vi "WriteI64.vi"(10 "Data":i64, 11 "Address":u32) -> ()   [LabVIEW 2016]
uses:
  <vilib>/rvi/Memory/Memory_Emulation/nirvimemoryFastEmulation.vi
  <vilib>/rvi/Memory/Memory_Emulation/nirvimemoryEmulation.vi
  <vilib>/rvi/Emulation/niFpgaEmulationIsFPGAContextNoSignature.vi
  <vilib>/rvi/DataTransferAndStorage/Container/Common/niFpgaContainerGetUniqueNameForEmu.vi
  <vilib>/rvi/Emulation/niFpgaProcessEmulError.vi
  <vilib>/rvi/Emulation/niFpgaSctlEmulationGetInTimedLoop.vi
  <vilib>/rvi/errors/nirviReportUnexpectedCaseInternalError (U32).vi
  <vilib>/rvi/DataTransferAndStorage/Container/Common/niFpgaContainerExecOnDevCompGetState.vi
  <vilib>/rvi/Memory/Memory_Emulation/niFpgaMemoryEmulationCacheClearOnFirstRun.vi
  <vilib>/rvi/Memory/Memory_Emulation/nirvimemoryEmulationManagerCache_MakeExclusive.vi
  <vilib>/rvi/Memory/Memory_Emulation/niFpgaMemoryEmulationValidateCache.vi
  <vilib>/rvi/Memory/Memory_Emulation/nirvimemoryEmulationManagerCache_InsertValue.vi
  <vilib>/Utility/error.llb/Clear Errors.vi
  <vilib>/rvi/Memory/Memory_Emulation/nirvimemoryEmulationManagerCache_ReleaseExclusive.vi
  <vilib>/rvi/Memory/Memory_Emulation/nirvimemoryEmulationManagerCache_GetValue.vi
  <vilib>/rvi/Memory/Memory_Emulation/nirvimemoryEmulationManagerCache_SetValue.vi
  <vilib>/rvi/Emulation/niFpgaSctlEmulationResourceMgr.vi
  <vilib>/rvi/DataTransferAndStorage/Container/XNode/niFpgaContainer.xnode
  <vilib>/rvi/Memory/Memory_Emulation/niFpgaMemoryEmulationRefIn.vi
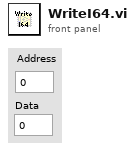
[diagram p1: front panel]
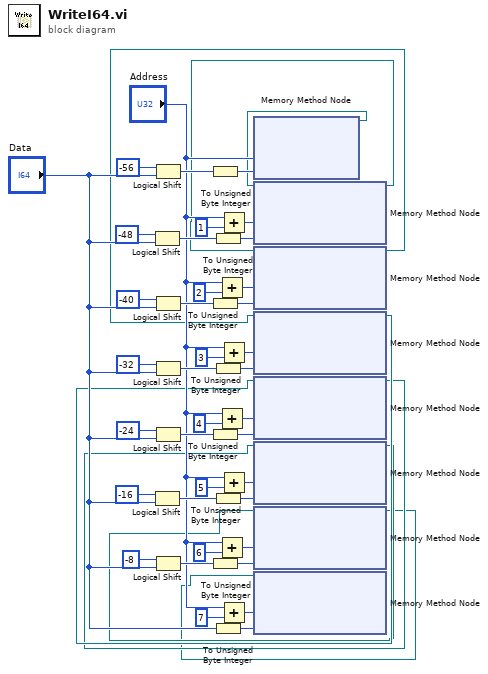
[diagram p0: block diagram]
diagram:
  n1 = Logical Shift(y=i16 -48, x="Data") -> (x << y=w30:i64)
  n2 = Logical Shift(y=i16 -16, x="Data") -> (x << y=w29:i64)
  n3 = Logical Shift(y=i16 -56, x="Data") -> (x << y=w41:i64)
  n4 = Logical Shift(y=i16 -40, x="Data") -> (x << y=w38:i64)
  n5 = Logical Shift(y=i16 -32, x="Data") -> (x << y=w12:i64)
  n6 = Logical Shift(y=i16 -24, x="Data") -> (x << y=w18:i64)
  n7 = Logical Shift(y=i16 -8, x="Data") -> (x << y=w21:i64)
  n8 = To Unsigned Byte Integer(number=w41) -> (unsigned 8bit integer=w42:u8)
  n9 = To Unsigned Byte Integer(number=w38) -> (unsigned 8bit integer=w37:u8)
  n10 = To Unsigned Byte Integer(number=w18) -> (unsigned 8bit integer=w17:u8)
  n11 = To Unsigned Byte Integer(number=w21) -> (unsigned 8bit integer=w22:u8)
  n12 = To Unsigned Byte Integer(number=w30) -> (unsigned 8bit integer=w40:u8)
  n13 = To Unsigned Byte Integer(number=w12) -> (unsigned 8bit integer=w39:u8)
  n14 = To Unsigned Byte Integer(number=w29) -> (unsigned 8bit integer=w19:u8)
  n15 = To Unsigned Byte Integer(number="Data") -> (unsigned 8bit integer=w20:u8)
  n16 = Add(x="Address", y=u32 2) -> (x+y=w32:u32)
  n17 = Add(x="Address", y=u32 4) -> (x+y=w10:u32)
  n18 = Add(x="Address", y=u32 6) -> (x+y=w27:u32)
  n19 = Add(x="Address", y=u32 1) -> (x+y=w45:u32)
  n20 = Add(x="Address", y=u32 3) -> (x+y=w34:u32)
  n21 = Add(x="Address", y=u32 5) -> (x+y=w14:u32)
  n22 = Add(x="Address", y=u32 7) -> (x+y=w25:u32)
  n23 = xnode ("Memory Method Node")("Address"="Address", "Data"=w42) -> ("Memory Out"=w7:refnum<k21>)  [unwired: 1 in]
  n24 = xnode ("Memory Method Node")("Address"=w45, "Data"=w40, "Memory In"=w7) -> ("Memory Out"=w6:refnum<k21>)
  n25 = xnode ("Memory Method Node")("Address"=w32, "Data"=w37, "Memory In"=w6) -> ("Memory Out"=w5:refnum<k21>)
  n26 = xnode ("Memory Method Node")("Address"=w34, "Data"=w39, "Memory In"=w5) -> ("Memory Out"=w4:refnum<k21>)
  n27 = xnode ("Memory Method Node")("Address"=w10, "Data"=w17, "Memory In"=w4) -> ("Memory Out"=w3:refnum<k21>)
  n28 = xnode ("Memory Method Node")("Address"=w14, "Data"=w19, "Memory In"=w3) -> ("Memory Out"=w2:refnum<k21>)
  n29 = xnode ("Memory Method Node")("Address"=w27, "Data"=w22, "Memory In"=w2) -> ("Memory Out"=w1:refnum<k21>)
  n30 = xnode ("Memory Method Node")("Address"=w25, "Data"=w20, "Memory In"=w1) -> ()  [unwired: 1 out]
